vi "Interporation (SubVI).vi"(2 "method":i32(ring)=1 caption="Method" items=["최근접", "선형", "스플라인", "3차 에르미트", "라그랑지"], 3 "Sample":i32, 4 "Y_long":dbl[](array[numeric]) format="%#_13g", 5 "X_lat":dbl[](array[numeric]) format="%#_13g") -> (0 "Y_long":dbl[](array[numeric]) format="%.6g", 1 "X_lat":dbl[](array[numeric]) format="%.6g")   [LabVIEW 2024]
uses:
  <vilib>/Analysis/1siggen.llb/Ramp Pattern by Delta.vi
  <vilib>/Utility/file.llb/Read Delimited Spreadsheet (DBL).vi
  <vilib>/gmath/NI_Gmath.lvlib
  <vilib>/Analysis/NI_AALBase.lvlib
panel:
  out "XY 그래프":cluster{"yi":dbl[], "yi":dbl[]}(graph)
  in  "Test Log File":path
  # "X값도 보간\nY값도 보간\nSample : Origin Data 사이 값 갯수"
  # "그래프 제거"
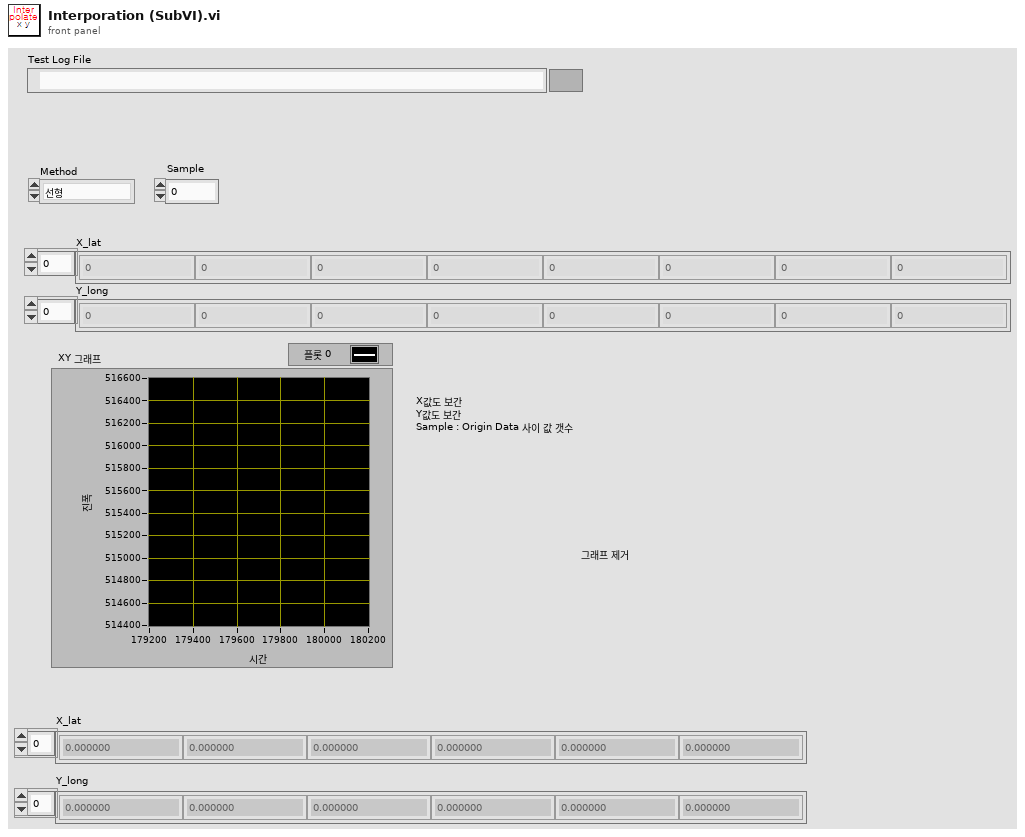
[diagram p1: front panel]
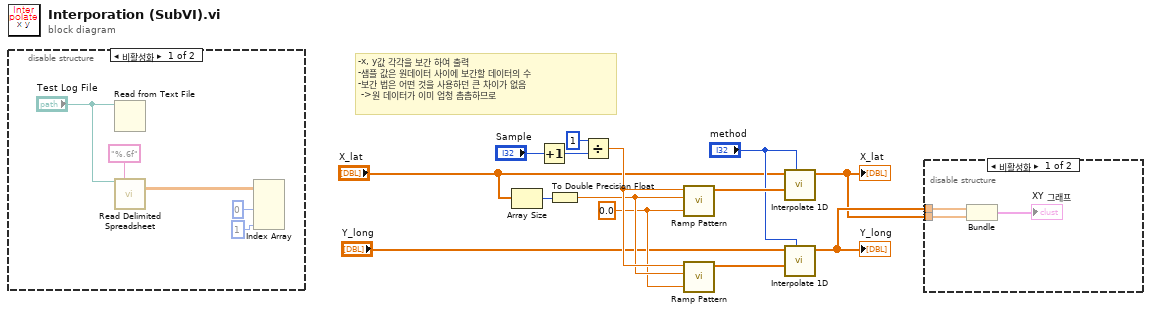
[diagram p0: block diagram]
diagram:
  w6 = 0.0 ("start")
  # "-x, y값 각각을 보간 하여 출력\n-샘플 값은 원데이터 사이에 보간할 데이터의 수\n-보간 법은 어떤 것을 사용하던 큰 차이가 없음 \n ->원 데이터가 이미 엄청 촘촘하므로"
  n1 = disable-structure shown="비활성화" {
    frame Disabled {
      n2 = Read from Text File(file (use dialog)="Test Log File") -> ()  [unwired: 3 in, 4 out]
      n3 = call-poly <vilib>:"Read Delimited Spreadsheet.vi"("file path (dialog if empty)"="Test Log File", "format (%.3f)"="%.6f") -> ("all rows"=w19:dbl[][])  [unwired: 8 in, 5 out]
      n4 = Index Array(array=w19, index (col) #1=0, index (col) #2=1 ("index (col)")) -> ()  [unwired: 2 in, 2 out]
    }
    frame Enabled {
    }
  }
  n5 = Array Size(array="X_lat") -> (size(s)=w14:i32)
  n6 = Increment(x="Sample") -> (x+1=w13:i32)
  n7 = To Double Precision Float(number=w14) -> (double precision float=w7:dbl)
  n8 = Divide(x=1, y=w13) -> (x/y=w8:dbl)
  n9 = call-poly <vilib>:"Ramp Pattern.vi"("start"=w6, "end"=w7, "delta"=w8) -> ("Ramp Pattern"=w10:dbl[])  [unwired: 6 in, 2 out]
  n10 = call-poly <vilib>:"Ramp Pattern.vi"("start"=w6, "end"=w7, "delta"=w8) -> ("Ramp Pattern"=w9:dbl[])  [unwired: 6 in, 2 out]
  n11 = call <vilib>:"Interpolate 1D.vi"("method"="method", "xi"=w10, "Y"="X_lat") -> ("yi"=w4:dbl[])  [unwired: 6 in, 2 out]
  "X_lat" <- w4
  n12 = call <vilib>:"Interpolate 1D.vi"("method"="method", "xi"=w9, "Y"="Y_long") -> ("yi"=w5:dbl[])  [unwired: 6 in, 2 out]
  "Y_long" <- w5
  n13 = disable-structure shown="비활성화" {
    disable-tunnel: w5 -> [w21 _]
    disable-tunnel: w4 -> [w20 _]
    frame Disabled {
      n14 = Bundle("yi"=w21, "yi"=w20) -> (→"XY 그래프":cluster{"yi":dbl[], "yi":dbl[]})  [unwired: 1 in]
    }
    frame Enabled {
    }
  }
